vi "Straight Drive.vi"(0 "Controller 1":T1={"Joystick 1 X"=0.0, "Joystick 1 Y"=0.0, "Joystick 2 Z"=0.0, "Joystick 2 Rotate"=1.0, "Button B"=FALSE}) -> (1 "Joystick X":dbl, 2 "Joystick Y":dbl, 3 "Joystick Z":dbl)   [LabVIEW 2016]
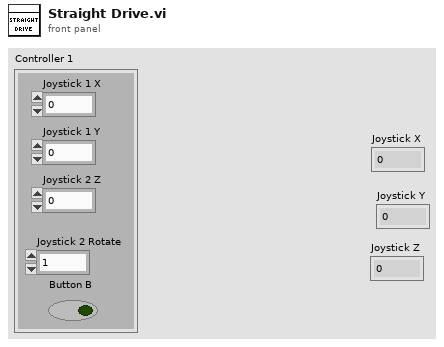
[diagram p1: front panel]
types:
  T1 = cluster{"Joystick 1 X":dbl, "Joystick 1 Y":dbl, "Joystick 2 Z":dbl, "Joystick 2 Rotate":dbl, "Button B":bool}
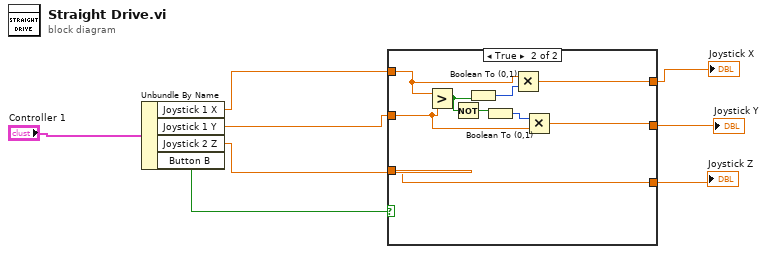
[diagram p0: block diagram]
diagram:
  n1 = Unbundle By Name("Controller 1") -> ("Joystick 1 X"=w5:dbl, "Joystick 1 Y"=w4:dbl, "Joystick 2 Z"=w3:dbl, "Button B"=w1:bool)
  n2 = case shown="True" w1 {
    tunnel: w5 -> [w11 w17]
    tunnel: w4 -> [w10 w12]
    tunnel: w3 -> [w9 w20]
    tunnel: [w11 w19] -> w8
    tunnel: [w9 w20] -> w7
    tunnel: [w10 w18] -> w6
    frame False {
    }
    frame True {
      n3 = Greater?(x=w17, y=w12) -> (0:w15:bool)
      n4 = Not(x=w15) -> (.not. x?=w14:bool)
      n5 = Boolean To (0,1)(Boolean=w15) -> (0, 1=w16:i16)
      n6 = Boolean To (0,1)(Boolean=w14) -> (0, 1=w13:i16)
      n7 = Multiply(x=w17, y=w16) -> (x*y=w19:dbl)
      n8 = Multiply(x=w13, y=w12) -> (x*y=w18:dbl)
    }
  }
  "Joystick X" <- w8
  "Joystick Y" <- w6
  "Joystick Z" <- w7
